vi "电源.vi"() -> ()   [LabVIEW 2021]
uses:
  <vilib>/Instr/_visa.llb/VISA Configure Serial Port (Instr).vi
  dec08355-b419-423e-8ff6-95b1478ea6fa.vi
panel:
  in  "电源串口":refnum<visa-resource-name>
  in  "单选按钮":enum32{"Item 0", "Item 1"}(radio)
  out "电源电压":dbl format="%#_6f V"
  out "电源电流":dbl format="%#_6f A"
  in  "设定电流":dbl format="%#_g A"
  in  "设定电流":bool
  out "状态":string
  out "磁铁端口":refnum<visa-resource-name> caption="VISA资源名称输出"
  in  "关闭电源":bool
  out "控制读取磁场":bool
  in  "启动电源":bool
  in  "设定磁场":dbl format="%#_g Gs"
  in  "设定磁场":bool
  in  "退磁":bool
  out "当前磁场":dbl format="%#_g Gs"
  in  "电流速率":dbl=10.0 format="%#_g (A/S)"
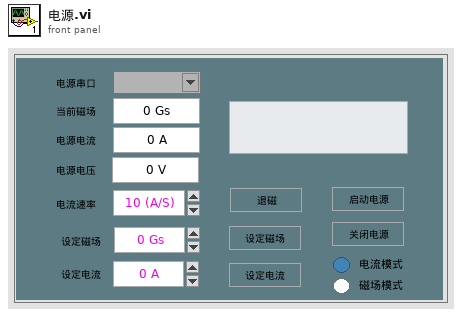
[diagram p1: front panel]
types:
  T1 = enum32{"Invalid", "Standard", "Closed", "Hidden", "Minimized", "Maximized"}
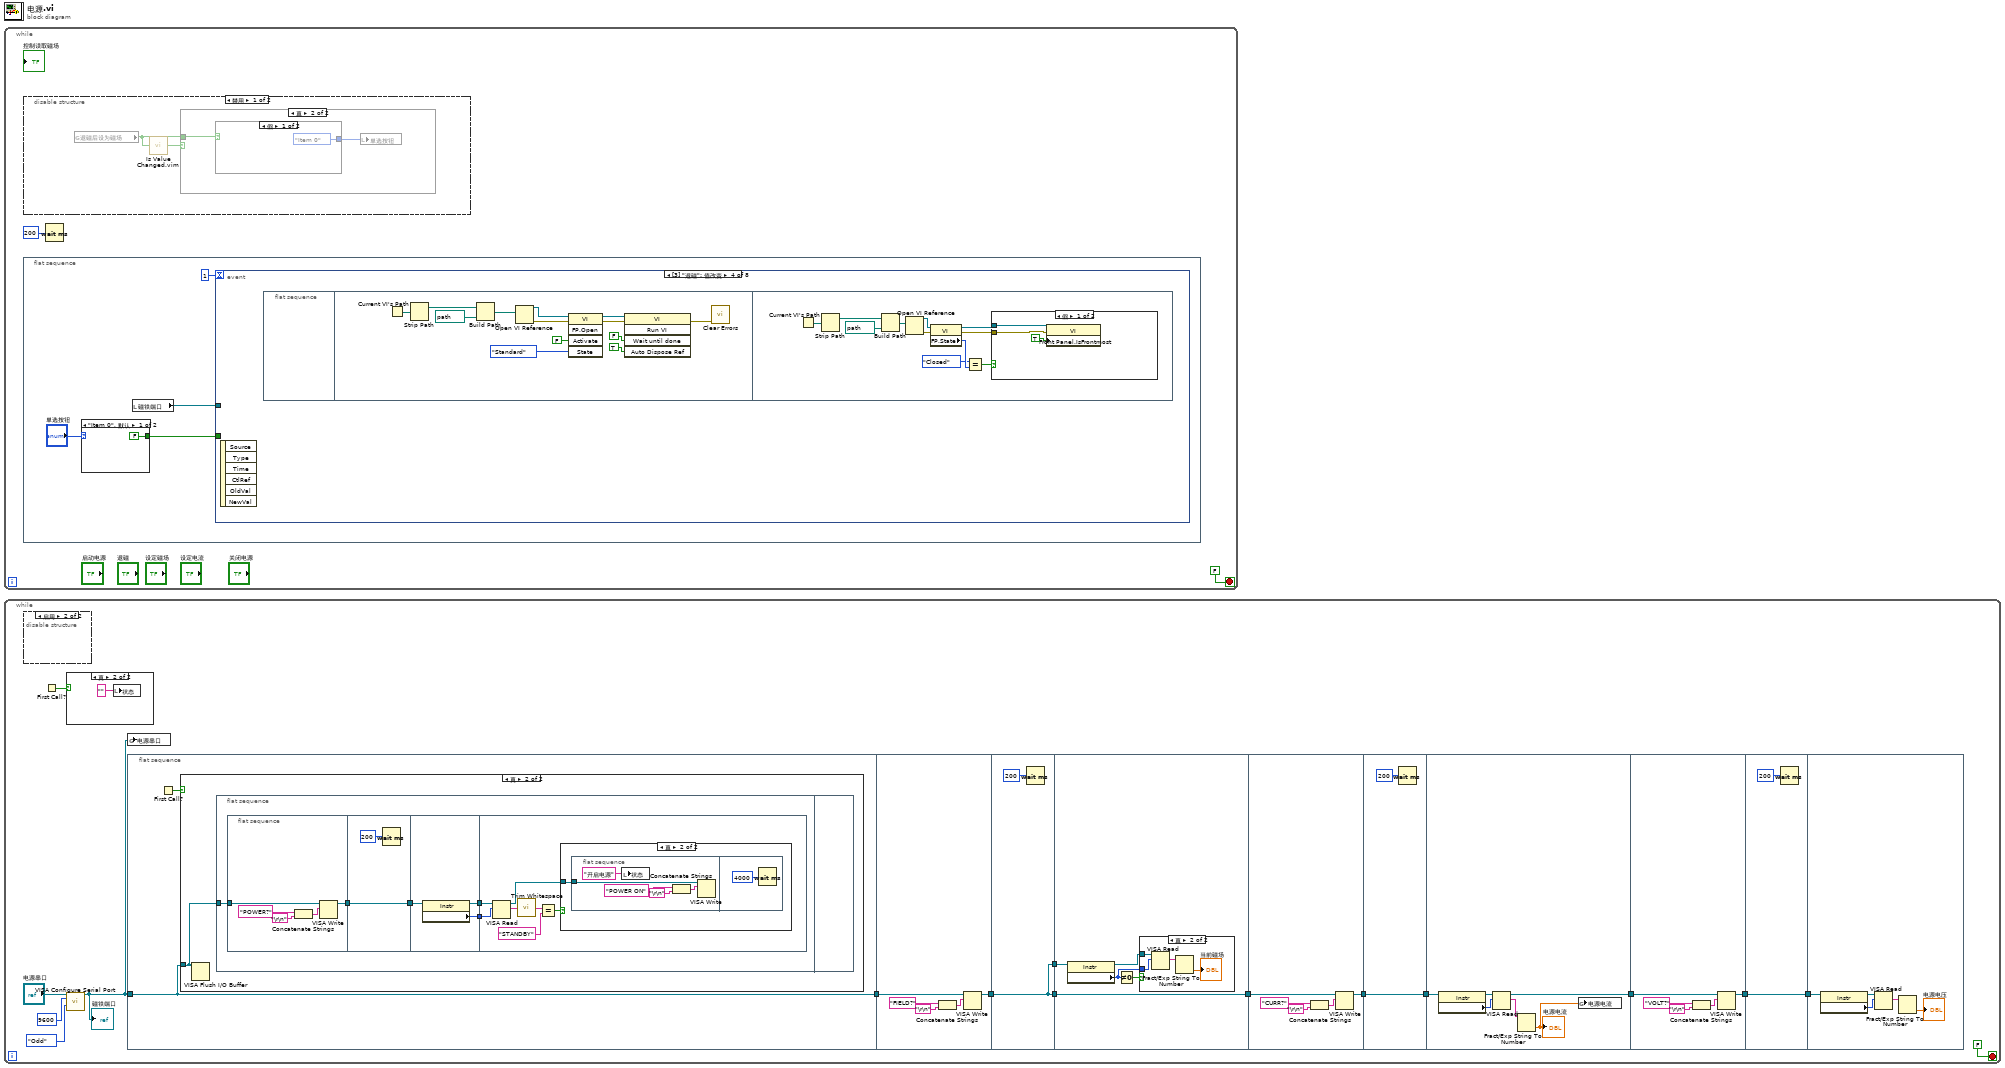
[diagram p0: block diagram]
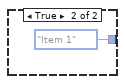
[diagram p3: hidden frame]
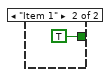
[diagram p5: hidden frame]
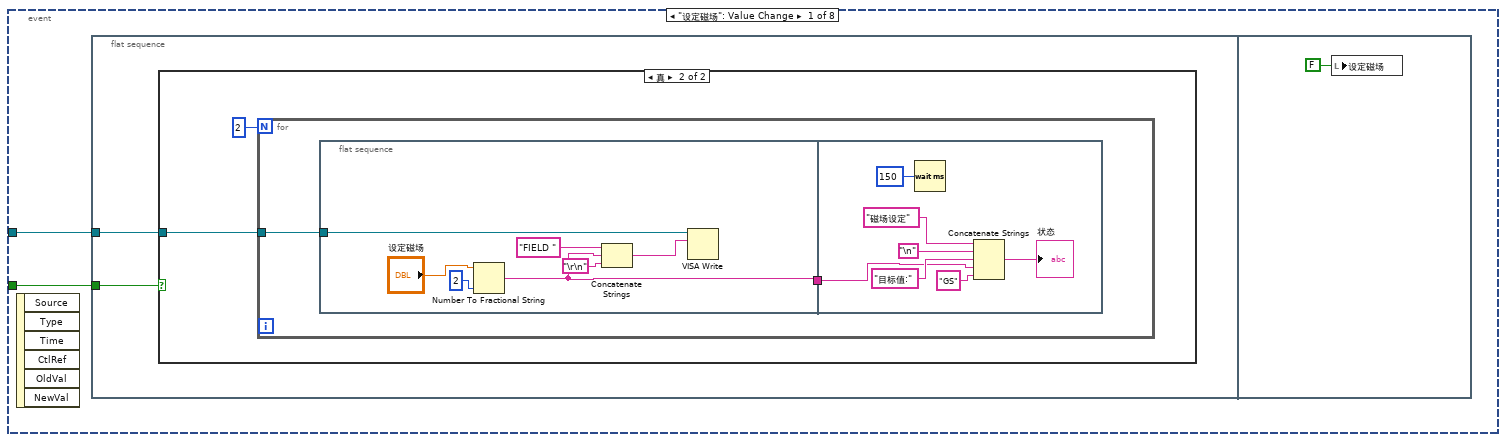
[diagram p6: hidden frame]
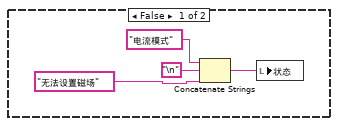
[diagram p7: hidden frame]
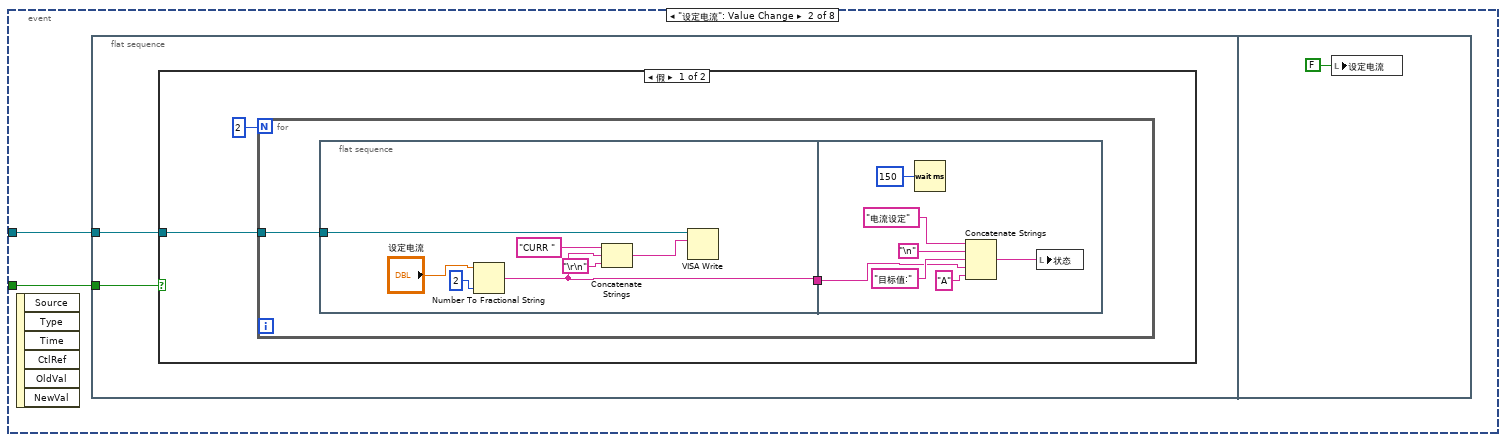
[diagram p8: hidden frame]
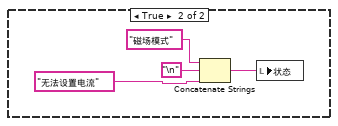
[diagram p9: hidden frame]
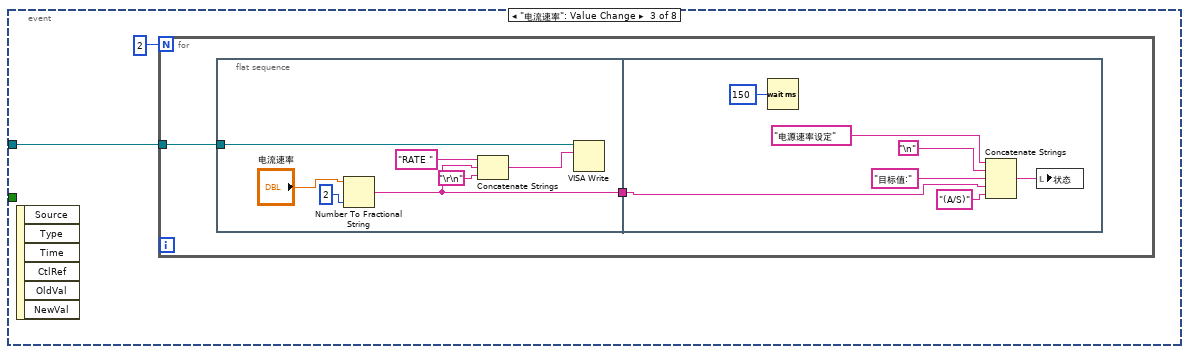
[diagram p10: hidden frame]
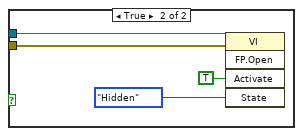
[diagram p11: hidden frame]
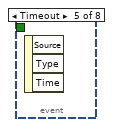
[diagram p12: hidden frame]
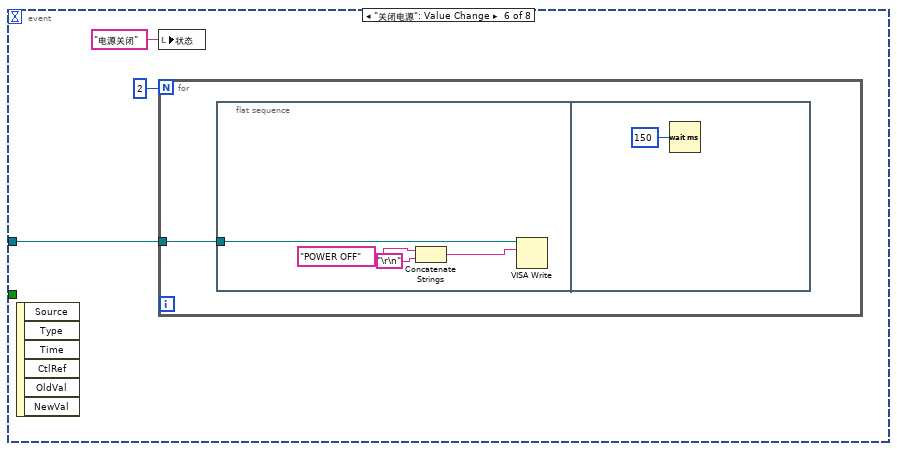
[diagram p13: hidden frame]
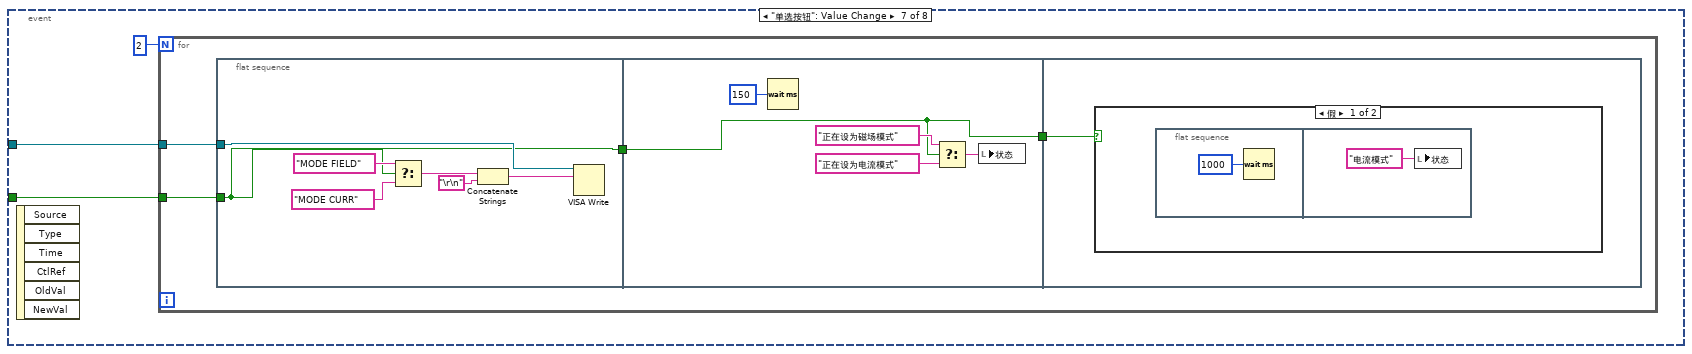
[diagram p14: hidden frame]
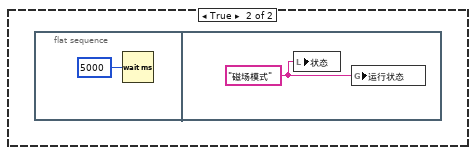
[diagram p15: hidden frame]
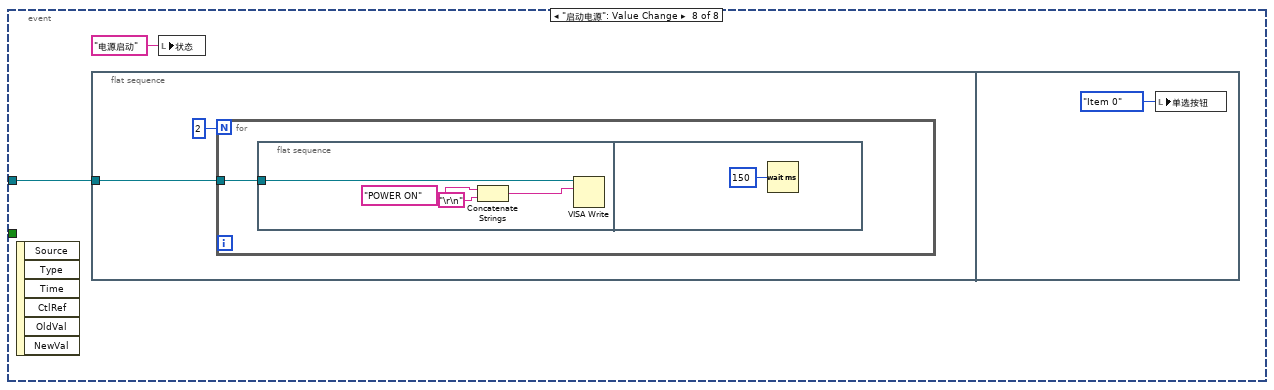
[diagram p16: hidden frame]
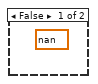
[diagram p19: hidden frame]
diagram:
  n1 = while {
    stop <- FALSE stop-if-true
    n2 = disable-structure shown="禁用" {
      frame Disabled {
        n3 = global read "退磁后设为磁场.vi" "退磁后设为磁场"() -> (w3:bool)
        n4 = call "Is Value Changed.vim"("value"=w3) -> ("changed or first call?"=w4:bool)
        n5 = case shown="真" w4 {
          tunnel: w3 -> [_ w6]
          frame False {
          }
          frame True {
            n6 = case shown="假" w6 {
              tunnel: [enum32{"Item 0", "Item 1"}."Item 0" ("单选按钮") enum32{"Item 0", "Item 1"}."Item 1" ("单选按钮")] -> w5
              frame False {
              }
              frame True {
              }
            }
            n7 = local write "单选按钮"(w5) -> ()
          }
        }
      }
      frame Enabled {
      }
    }
    n8 = flat-sequence {
      frame #0 {
        n9 = case shown="\"Item 0\", 默认" "单选按钮" {
          tunnel: [FALSE TRUE] -> w9
          frame "Item 0", Default {
          }
          frame "Item 1" {
          }
        }
        n10 = local read "磁铁端口"() -> (w11:refnum<visa-resource-name>)
        n11 = event shown="[3] \"退磁\": 值改变" {
          selector: _ -> [_ _ _ _ _ _ _ _]
          dyn-events: _ -> [_ _ _ _ _ _ _ _]
          timeout: 1 -> [_ _ _ _ _ _ _ _]
          tunnel: w11 -> [w16 w43 w70 _ _ w120 w128 w152]
          tunnel: w9 -> [w15 w42 _ _ _ _ w129 _]
          event "设定磁场": Value Change {
            n12 = event-data() -> ()  [unwired: 1 in, 6 out]
            n13 = flat-sequence {
              tunnel: w16 -> [w18]
              tunnel: w15 -> [w17]
              frame #0 {
                n14 = case shown="真" w17 {
                  tunnel: w18 -> [_ w23]
                  frame False {
                    n15 = Concatenate Strings("电流模式" ("字符串"), "\n", "无法设置磁场" ("字符串")) -> (w22:string)
                    n16 = local write "状态"(w22) -> ()
                  }
                  frame True {
                    n17 = for {
                      N: 2 -> [_]
                      tunnel: w23 -> [w26]
                      n18 = flat-sequence {
                        tunnel: w26 -> [w31]
                        tunnel: [w27] -> w25
                        tunnel: w25 -> [w35]
                        frame #0 {
                          n19 = Number To Fractional String(number="设定磁场", precision (6)=i16 2 ("精度(6)")) -> (F-format string=w27:string)  [unwired: 2 in]
                          n20 = Concatenate Strings("FIELD " ("字符串"), w27, "\r\n") -> (w33:string)
                          n21 = VISA Write(VISA resource name=w31, write buffer=w33) -> ()  [unwired: 1 in, 3 out]
                        }
                        frame #1 {
                          n22 = Wait (ms)(milliseconds to wait=u32 150 ("等待时间（毫秒）")) -> ()  [unwired: 1 out]
                          n23 = Concatenate Strings("磁场设定" ("字符串"), "\n", "目标值:" ("字符串"), w35, "GS" ("字符串")) -> (→"状态":string)
                        }
                      }
                    }
                  }
                }
              }
              frame #1 {
                n24 = local write "设定磁场"(FALSE ("设定磁场")) -> ()
              }
            }
          }
          event "设定电流": Value Change {
            n25 = event-data() -> ()  [unwired: 1 in, 6 out]
            n26 = flat-sequence {
              tunnel: w43 -> [w45]
              tunnel: w42 -> [w44]
              frame #0 {
                n27 = case shown="假" w44 {
                  tunnel: w45 -> [w46 _]
                  frame False {
                    n28 = for {
                      N: 2 -> [_]
                      tunnel: w46 -> [w49]
                      n29 = flat-sequence {
                        tunnel: w49 -> [w54]
                        tunnel: [w50] -> w48
                        tunnel: w48 -> [w58]
                        frame #0 {
                          n30 = Number To Fractional String(number="设定电流", precision (6)=i16 2 ("精度(6)")) -> (F-format string=w50:string)  [unwired: 2 in]
                          n31 = Concatenate Strings("CURR " ("字符串"), w50, "\r\n") -> (w56:string)
                          n32 = VISA Write(VISA resource name=w54, write buffer=w56) -> ()  [unwired: 1 in, 3 out]
                        }
                        frame #1 {
                          n33 = Wait (ms)(milliseconds to wait=u32 150 ("等待时间（毫秒）")) -> ()  [unwired: 1 out]
                          n34 = Concatenate Strings("电流设定" ("字符串"), "\n", "目标值:" ("字符串"), w58, "A" ("字符串")) -> (w57:string)
                          n35 = local write "状态"(w57) -> ()
                        }
                      }
                    }
                  }
                  frame True {
                    n36 = Concatenate Strings("磁场模式" ("字符串"), "\n", "无法设置电流" ("字符串")) -> (w67:string)
                    n37 = local write "状态"(w67) -> ()
                  }
                }
              }
              frame #1 {
                n38 = local write "设定电流"(FALSE ("设定电流")) -> ()
              }
            }
          }
          event "电流速率": Value Change {
            n39 = event-data() -> ()  [unwired: 1 in, 6 out]
            n40 = for {
              N: 2 -> [_]
              tunnel: w70 -> [w72]
              n41 = flat-sequence {
                tunnel: w72 -> [w77]
                tunnel: [w74] -> w71
                tunnel: w71 -> [w80]
                frame #0 {
                  n42 = Number To Fractional String(number="电流速率", precision (6)=i16 2 ("精度(6)")) -> (F-format string=w74:string)  [unwired: 2 in]
                  n43 = Concatenate Strings("RATE " ("字符串"), w74, "\r\n") -> (w79:string)
                  n44 = VISA Write(VISA resource name=w77, write buffer=w79) -> ()  [unwired: 1 in, 3 out]
                }
                frame #1 {
                  n45 = Wait (ms)(milliseconds to wait=u32 150 ("等待时间（毫秒）")) -> ()  [unwired: 1 out]
                  n46 = Concatenate Strings("电源速率设定" ("字符串"), "\n", "目标值:" ("字符串"), w80, "(A/S)" ("字符串")) -> (w85:string)
                  n47 = local write "状态"(w85) -> ()
                }
              }
            }
          }
          event "退磁": Value Change {
            n48 = event-data() -> ()  [unwired: 1 in, 6 out]
            n49 = flat-sequence {
              frame #0 {
              }
              frame #1 {
                n50 = Current VI's Path() -> (path=w99:path)
                n51 = Strip Path(path=w99) -> (stripped path=w98:path)  [unwired: 1 out]
                n52 = Build Path(base path=w98, name or relative path=path "退磁.vi" ("名称或相对路径")) -> (appended path=w97:path)
                n53 = Open VI Reference(vi path=w97) -> (vi reference=w95:refnum<vi>, error out=w93:errorcluster)  [unwired: 5 in]
                n54 = invoke class="VI" method="FP.Open"(reference=w95, error in=w93, "Activate"=FALSE ("激活？"), "State"=T1."Standard" ("状态")) -> (reference out=w94:refnum<vi>, error out=w92:errorcluster)  [unwired: 1 in, 3 out]
                n55 = invoke class="VI" method="Run VI"(reference=w94, error in=w92, "Wait until done"=FALSE ("结束前等待"), "Auto Dispose Ref"=TRUE ("自动销毁引用")) -> (error out=w87:errorcluster)  [unwired: 1 in, 4 out]
                n56 = call <vilib>:"Clear Errors.vi"("error in (no error)"=w87) -> ()  [unwired: 5 in, 2 out]
              }
              frame #2 {
                n57 = Current VI's Path() -> (path=w101:path)
                n58 = Strip Path(path=w101) -> (stripped path=w100:path)  [unwired: 1 out]
                n59 = Build Path(base path=w100, name or relative path=path "退磁.vi" ("名称或相对路径")) -> (appended path=w110:path)
                n60 = Open VI Reference(vi path=w110) -> (vi reference=w104:refnum<vi>, error out=w105:errorcluster)  [unwired: 5 in]
                n61 = property class="VI"(reference=w104, error in=w105) -> (reference out=w108:refnum<vi>, error out=w109:errorcluster, "FP.State"=w106:T1)
                n62 = Equal?(x=T1."Closed" ("前面板窗口:状态"), y=w106) -> (x = y?=w107:bool)
                n63 = case shown="假" w107 {
                  tunnel: w108 -> [w112 w117]
                  tunnel: w109 -> [w111 w116]
                  frame False {
                    n64 = property class="VI"(reference=w112, error in=w111, "Front Panel.IsFrontmost"=TRUE ("前面板窗口:在最前")) -> ()  [unwired: 2 out]
                  }
                  frame True {
                    n65 = invoke class="VI" method="FP.Open"(reference=w117, error in=w116, "Activate"=TRUE ("激活？"), "State"=T1."Hidden" ("状态")) -> ()  [unwired: 1 in, 5 out]
                  }
                }
              }
            }
          }
          event Timeout {
            n66 = event-data() -> ()  [unwired: 1 in, 3 out]
          }
          event "关闭电源": Value Change {
            n67 = event-data() -> ()  [unwired: 1 in, 6 out]
            n68 = local write "状态"("电源关闭" ("字符串")) -> ()
            n69 = for {
              N: 2 -> [_]
              tunnel: w120 -> [w121]
              n70 = flat-sequence {
                tunnel: w121 -> [w125]
                frame #0 {
                  n71 = Concatenate Strings("POWER OFF", "\r\n") -> (w122:string)
                  n72 = VISA Write(VISA resource name=w125, write buffer=w122) -> ()  [unwired: 1 in, 3 out]
                }
                frame #1 {
                  n73 = Wait (ms)(milliseconds to wait=u32 150 ("等待时间（毫秒）")) -> ()  [unwired: 1 out]
                }
              }
            }
          }
          event "单选按钮": Value Change {
            n74 = event-data() -> ()  [unwired: 1 in, 6 out]
            n75 = for {
              N: 2 -> [_]
              tunnel: w129 -> [w133]
              tunnel: w128 -> [w132]
              n76 = flat-sequence {
                tunnel: w133 -> [w134]
                tunnel: w132 -> [w135]
                tunnel: [w134] -> w131
                tunnel: w131 -> [w141]
                tunnel: [w141] -> w130
                tunnel: w130 -> [w146]
                frame #0 {
                  n77 = Select(t="MODE FIELD", s=w134, f="MODE CURR") -> (s? t:f=w140:string)
                  n78 = Concatenate Strings(w140, "\r\n") -> (w139:string)
                  n79 = VISA Write(VISA resource name=w135, write buffer=w139) -> ()  [unwired: 1 in, 3 out]
                }
                frame #1 {
                  n80 = Wait (ms)(milliseconds to wait=u32 150 ("等待时间（毫秒）")) -> ()  [unwired: 1 out]
                  n81 = Select(t="正在设为磁场模式", s=w141, f="正在设为电流模式") -> (s? t:f=w142:string)
                  n82 = local write "状态"(w142) -> ()
                }
                frame #2 {
                  n83 = case shown="假" w146 {
                    frame False {
                      n84 = flat-sequence {
                        frame #0 {
                          n85 = Wait (ms)(milliseconds to wait=u32 1000 ("等待时间（毫秒）")) -> ()  [unwired: 1 out]
                        }
                        frame #1 {
                          n86 = local write "状态"("电流模式" ("f")) -> ()
                        }
                      }
                    }
                    frame True {
                      n87 = flat-sequence {
                        frame #0 {
                          n88 = Wait (ms)(milliseconds to wait=u32 5000 ("等待时间（毫秒）")) -> ()  [unwired: 1 out]
                        }
                        frame #1 {
                          w150 = "磁场模式"
                          n89 = local write "状态"(w150) -> ()
                          n90 = global write "运行状态.vi" "运行状态"(w150) -> ()
                        }
                      }
                    }
                  }
                }
              }
            }
          }
          event "启动电源": Value Change {
            n91 = event-data() -> ()  [unwired: 1 in, 6 out]
            n92 = flat-sequence {
              tunnel: w152 -> [w154]
              frame #0 {
                n93 = for {
                  N: 2 -> [_]
                  tunnel: w154 -> [w155]
                  n94 = flat-sequence {
                    tunnel: w155 -> [w159]
                    frame #0 {
                      n95 = Concatenate Strings("POWER ON", "\r\n") -> (w156:string)
                      n96 = VISA Write(VISA resource name=w159, write buffer=w156) -> ()  [unwired: 1 in, 3 out]
                    }
                    frame #1 {
                      n97 = Wait (ms)(milliseconds to wait=u32 150 ("等待时间（毫秒）")) -> ()  [unwired: 1 out]
                    }
                  }
                }
              }
              frame #1 {
                n98 = local write "单选按钮"(enum32{"Item 0", "Item 1"}."Item 0" ("单选按钮")) -> ()
              }
            }
            n99 = local write "状态"("电源启动" ("字符串")) -> ()
          }
        }
      }
    }
    n100 = Wait (ms)(milliseconds to wait=u32 200 ("等待时间（毫秒）")) -> ()  [unwired: 1 out]
  }
  n101 = while {
    stop <- FALSE stop-if-true
    n102 = disable-structure shown="启用" {
      frame Disabled {
      }
      frame Enabled {
      }
    }
    n103 = First Call?() -> (First Call?: T/F=w176:bool)
    n104 = case shown="真" w176 {
      frame False {
      }
      frame True {
        n105 = local write "状态"("" ("状态")) -> ()
      }
    }
    n106 = call-poly "VISA Configure Serial Port"("VISA resource name"="电源串口", "baud rate (9600)"=u32 9600, "parity (0:none)"=enum16{"None", "Odd", "Even", "Mark", "Space"}."Odd") -> ("VISA resource name out"=w162:refnum<visa-resource-name>)  [unwired: 11 in, 1 out]
    "磁铁端口" <- w162
    n107 = global write "电源串口.vi" "电源串口"(w162) -> ()
    n108 = flat-sequence {
      tunnel: w162 -> [w178]
      tunnel: [w178] -> w175
      tunnel: [w214] -> w174
      tunnel: w175 -> [w213]
      tunnel: [w215] -> w173
      tunnel: w174 -> [w215]
      tunnel: [w215] -> w170
      tunnel: w173 -> [w221]
      tunnel: w170 -> [w217]
      tunnel: [w217] -> w169
      tunnel: w169 -> [w227]
      tunnel: [w226] -> w167
      tunnel: [w231] -> w168
      tunnel: w167 -> [w231]
      tunnel: w168 -> [w238]
      tunnel: [w234] -> w166
      tunnel: w166 -> [w241]
      tunnel: [w239] -> w164
      tunnel: [w245] -> w165
      tunnel: w164 -> [w245]
      tunnel: w165 -> [w247]
      frame #0 {
        n109 = First Call?() -> (First Call?: T/F=w179:bool)
        n110 = case shown="真" w179 {
          tunnel: w178 -> [_ w180]
          frame False {
          }
          frame True {
            n111 = VISA Flush I/O Buffer(VISA resource name=w180) -> ()  [unwired: 2 in, 2 out]
            n112 = flat-sequence {
              tunnel: w180 -> [w185]
              frame #0 {
                n113 = flat-sequence {
                  tunnel: w185 -> [w187]
                  tunnel: [w186] -> w184
                  tunnel: w184 -> [w191]
                  tunnel: [w191] -> w183
                  tunnel: w183 -> [w195]
                  tunnel: [w194] -> w182
                  tunnel: [w193] -> w181
                  tunnel: w182 -> [w202]
                  tunnel: w181 -> [w201]
                  frame #0 {
                    n114 = Concatenate Strings("POWER?" ("字符串"), "\r\n") -> (w190:string)
                    n115 = VISA Write(VISA resource name=w187, write buffer=w190) -> (VISA resource name out=w186:refnum<visa-resource-name>)  [unwired: 1 in, 2 out]
                  }
                  frame #1 {
                    n116 = Wait (ms)(milliseconds to wait=u32 200 ("等待时间（毫秒）")) -> ()  [unwired: 1 out]
                  }
                  frame #2 {
                    n117 = property class="Instr"(reference=w195) -> (reference out=w193:refnum<visa-resource-name>, "Serial Settings:Number of Bytes at Serial Port"=w194:u32)  [unwired: 1 in, 1 out]
                  }
                  frame #3 {
                    n118 = VISA Read(VISA resource name=w201, byte count=w202) -> (VISA resource name out=w196:refnum<visa-resource-name>, read buffer=w200:string)  [unwired: 1 in, 2 out]
                    n119 = call <vilib>:"Trim Whitespace.vi"("string"=w200) -> ("trimmed string"=w199:string)  [unwired: 1 in]
                    n120 = Equal?(x=w199, y="STANDBY") -> (x = y?=w197:bool)
                    n121 = case shown="真" w197 {
                      tunnel: w196 -> [_ w203]
                      frame False {
                      }
                      frame True {
                        n122 = flat-sequence {
                          tunnel: w203 -> [w205]
                          frame #0 {
                            n123 = local write "状态"("开启电源" ("字符串")) -> ()
                            n124 = Concatenate Strings("POWER ON" ("字符串"), "\r\n") -> (w208:string)
                            n125 = VISA Write(VISA resource name=w205, write buffer=w208) -> ()  [unwired: 1 in, 3 out]
                          }
                          frame #1 {
                            n126 = Wait (ms)(milliseconds to wait=u32 4000 ("等待时间（毫秒）")) -> ()  [unwired: 1 out]
                          }
                        }
                      }
                    }
                  }
                }
              }
              frame #1 {
              }
            }
          }
        }
      }
      frame #1 {
        n127 = Concatenate Strings("FIELD?" ("写入缓冲区"), "\r\n") -> (w210:string)
        n128 = VISA Write(VISA resource name=w213, write buffer=w210) -> (VISA resource name out=w214:refnum<visa-resource-name>)  [unwired: 1 in, 2 out]
      }
      frame #2 {
        n129 = Wait (ms)(milliseconds to wait=u32 200 ("等待时间（毫秒）")) -> ()  [unwired: 1 out]
      }
      frame #3 {
        n130 = property class="Instr"(reference=w221) -> (reference out=w218:refnum<visa-resource-name>, "Serial Settings:Number of Bytes at Serial Port"=w219:u32)  [unwired: 1 in, 1 out]
        n131 = Not Equal To 0?(x=w219) -> (x != 0?=w220:bool)
        n132 = case shown="真" w220 {
          tunnel: w219 -> [_ w225]
          tunnel: w218 -> [_ w223]
          frame False {
            (unwired) nan
          }
          frame True {
            n133 = VISA Read(VISA resource name=w223, byte count=w225) -> (read buffer=w224:string)  [unwired: 1 in, 3 out]
            n134 = Fract/Exp String To Number(string=w224) -> (number=→"当前磁场":dbl)  [unwired: 3 in, 1 out]
          }
        }
      }
      frame #4 {
        n135 = Concatenate Strings("CURR?" ("写入缓冲区"), "\r\n") -> (w228:string)
        n136 = VISA Write(VISA resource name=w227, write buffer=w228) -> (VISA resource name out=w226:refnum<visa-resource-name>)  [unwired: 1 in, 2 out]
      }
      frame #5 {
        n137 = Wait (ms)(milliseconds to wait=u32 200 ("等待时间（毫秒）")) -> ()  [unwired: 1 out]
      }
      frame #6 {
        n138 = property class="Instr"(reference=w238) -> (reference out=w237:refnum<visa-resource-name>, "Serial Settings:Number of Bytes at Serial Port"=w236:u32)  [unwired: 1 in, 1 out]
        n139 = VISA Read(VISA resource name=w237, byte count=w236) -> (VISA resource name out=w234:refnum<visa-resource-name>, read buffer=w235:string)  [unwired: 1 in, 2 out]
        n140 = Fract/Exp String To Number(string=w235) -> (number=w233:dbl)  [unwired: 3 in, 1 out]
        "电源电流" <- w233
        n141 = global write "电流值.vi" "电源电流"(w233) -> ()
      }
      frame #7 {
        n142 = Concatenate Strings("VOLT?" ("字符串"), "\r\n") -> (w242:string)
        n143 = VISA Write(VISA resource name=w241, write buffer=w242) -> (VISA resource name out=w239:refnum<visa-resource-name>)  [unwired: 1 in, 2 out]
      }
      frame #8 {
        n144 = Wait (ms)(milliseconds to wait=u32 200 ("等待时间（毫秒）")) -> ()  [unwired: 1 out]
      }
      frame #9 {
        n145 = property class="Instr"(reference=w247) -> (reference out=w248:refnum<visa-resource-name>, "Serial Settings:Number of Bytes at Serial Port"=w249:u32)  [unwired: 1 in, 1 out]
        n146 = VISA Read(VISA resource name=w248, byte count=w249) -> (read buffer=w250:string)  [unwired: 1 in, 3 out]
        n147 = Fract/Exp String To Number(string=w250) -> (number=→"电源电压":dbl)  [unwired: 3 in, 1 out]
      }
    }
  }
